vi "niRFUtil LCAPI Copy 1D Array (1 I32, 3 DBL).vi"(0 "Source0 1D Array (I32)":i32[](array[numeric]), 5 "Source1 1D Array (DBL)":dbl[](array[numeric]) format="%.2f", 7 "Source2 1D Array (DBL)":dbl[](array[numeric]) format="%.2f", 9 "Source3 1D Array (DBL)":dbl[](array[numeric]) format="%.2f", 11 "error in (no error)":errorcluster, 12 "Data Copy Descriptor":u64) -> (4 "Source0 Out":i32[](array[numeric]), 6 "Source1 Out":dbl[](array[numeric]) format="%.2f", 8 "Source2 Out":dbl[](array[numeric]) format="%.2f", 10 "Source3 Out":dbl[](array[numeric]) format="%.2f", 15 "error out":errorcluster)   [LabVIEW 2015, in "niRFUtil.lvlib"]
uses:
  niRFUtil.lvlib
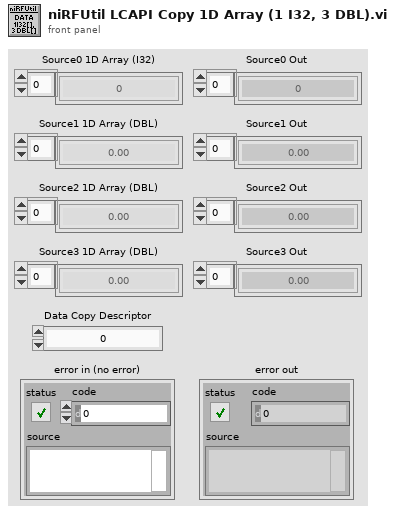
[diagram p1: front panel]
types:
  T1 = cluster{"status":bool, "return type":i32, "errorString":string}
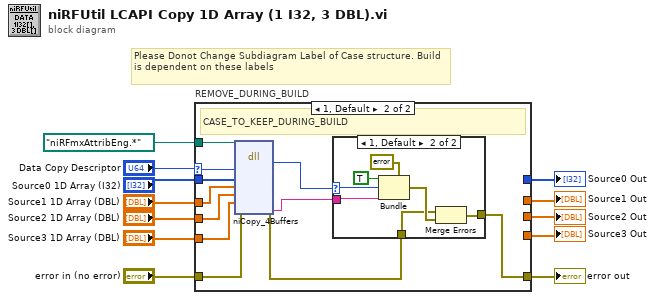
[diagram p0: block diagram]
diagram:
  # "Please Donot Change Subdiagram Label of Case structure. Build is dependent on these labels"
  n1 = case "REMOVE_DURING_BUILD" shown="1, Default" "Data Copy Descriptor" {
    selector: "Data Copy Descriptor" -> [_ w19]
    tunnel: "error in (no error)" -> [w13 w27]
    tunnel: "Source1 1D Array (DBL)" -> [w16 w26]
    tunnel: "Source2 1D Array (DBL)" -> [w15 w25]
    tunnel: "Source3 1D Array (DBL)" -> [w14 w24]
    tunnel: "Source0 1D Array (I32)" -> [w17 w23]
    tunnel: [w17 _] -> w4
    tunnel: [w16 _] -> w6
    tunnel: [w15 _] -> w3
    tunnel: [w14 _] -> w5
    tunnel: [w13 w28] -> w2
    tunnel: path "niRFmxAttribEng.*" ("path in") -> [_ w18]
    frame 0 {
      # "Development"
    }
    frame 1, Default {
      # "CASE_TO_KEEP_DURING_BUILD"
      n2 = dll-call lib="niRFmxAttribEng.*" fn="niCopy_4Buffers"(path in=w18, error in=w27, "dataCopyDescriptor"=w19, "source0"=w23, "source1"=w26, "source2"=w25, "source3"=w24) -> (error out=w20:errorcluster, "return type"=w22:i32, "errorString"=w21:string)  [unwired: 7 in, 1 out]
      n3 = case shown="1, Default" w22 {
        selector: w22 -> [_ w35]
        tunnel: w21 -> [_ w34]
        tunnel: w20 -> [w29 w30]
        tunnel: [w29 w33] -> w28
        frame 0 {
        }
        frame 1, Default {
          n4 = Bundle(cluster=T1 {"status"=FALSE, "return type"=0, "errorString"=""}, "status"=TRUE, "return type"=w35, "errorString"=w34) -> (w32:T1)
          n5 = Merge Errors(w30, w32) -> (w33:errorcluster)
        }
      }
    }
  }
  "error out" <- w2
  "Source0 Out" <- w4
  "Source1 Out" <- w6
  "Source2 Out" <- w3
  "Source3 Out" <- w5
